vi "onReadPlatanoConfiguration.vi"(7 "Section (default)":string, 8 "error in (no error)":errorcluster, 10 "Config Map in":map{string, string}(c390), 11 "Platano.CarayaTestSuite in":refnum<class "Platano.CarayaTestSuite.lvclass">) -> (0 "error out":errorcluster, 2 "Config Map out":map{string, string}(c390), 3 "Platano.CarayaTestSuite out":refnum<class "Platano.CarayaTestSuite.lvclass">)   [LabVIEW 2021, in "Banana.Caraya.lvlib" / "Platano.CarayaTestSuite.lvclass"]
uses:
  Platano.CarayaTestSuite.lvclass
  Bananas/Platano/Platano.lvclass
  Platano.CarayaTestSuite.lvclass/Platano.CarayaTestSuite.ctl
  <vilib>/addons/_JKI Toolkits/Caraya/classes/Properties/Properties.lvclass/Properties.ctl
  <vilib>/addons/_JKI Toolkits/Caraya/classes/Properties.Suite/Properties.Suite.lvclass
  C:/Program Files (x86)/National Instruments/LabVIEW 2021/vi.lib/addons/_JKI Toolkits/Caraya/classes/Properties/Properties.lvclass
  <vilib>/addons/_JKI Toolkits/Caraya/classes/Properties/Properties.lvclass
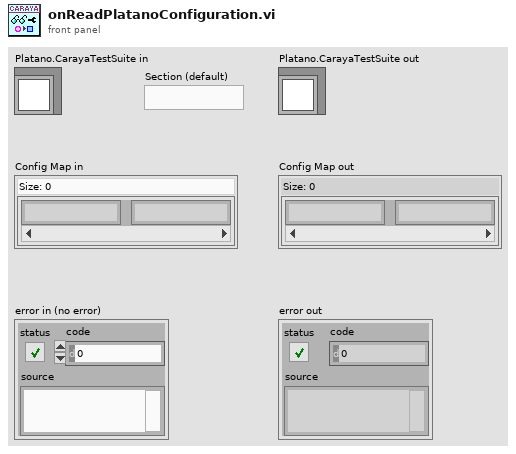
[diagram p1: front panel]
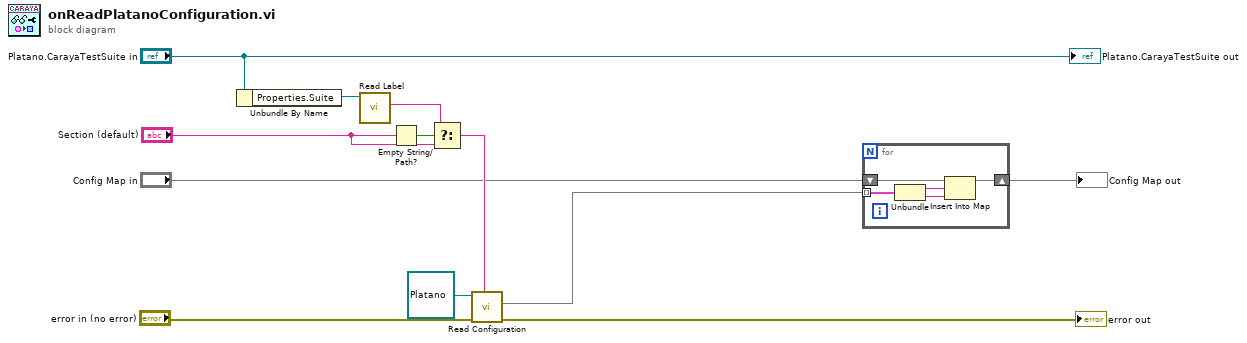
[diagram p0: block diagram]
diagram:
  n1 = Unbundle By Name("Platano.CarayaTestSuite in") -> ("Properties.Suite"=w11:refnum<class "Properties.Suite.lvclass">)
  n2 = call <vilib>:"Read Label.vi"("Properties in"=w11) -> ("Test Label"=w7:string)  [unwired: 9 in, 1 out]
  n3 = Empty String/Path?(string/path="Section (default)") -> (empty?=w8:bool)
  n4 = Select(t=w7, s=w8, f="Section (default)") -> (s? t:f=w6:string)
  n5 = call "Read Configuration.vi"("Section (default)"=w6, "error in (no error)"="error in (no error)", "Platano in"=refnum<class "Platano.lvclass"> refnum) -> ("error out"=→"error out":errorcluster, "Config Map"=w2:map{string, string})  [unwired: 6 in, 1 out]
  n6 = for {
    tunnel: w2 -> [w17] mode=indexing
    shift-right: [w13] -> w3
    shift-left: "Config Map in" -> [w16]
    n7 = Unbundle(w17) -> ("key"=w15:string, "value"=w14:string)
    n8 = Insert Into Map(map in=w16, key=w15, value=w14) -> (map out=w13:map{string, string})  [unwired: 2 out]
  }
  "Config Map out" <- w3
  "Platano.CarayaTestSuite out" <- "Platano.CarayaTestSuite in"
